vi "GetShiftTime.vi"(8 "error in (no error)":errorcluster, 11 "Time":timestamp) -> (0 "error out":errorcluster, 1 "Shift Elapsed Time [s]":dbl, 2 "Shift Start Time":timestamp, 3 "Shift End Time":timestamp)   [LabVIEW 2016]
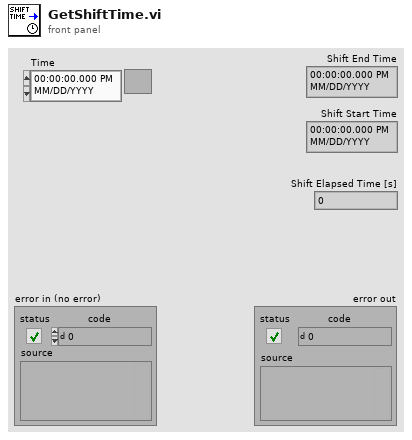
[diagram p1: front panel]
types:
  T1 = typedef "LVDateTimeRec.ctl" = cluster{"fractional second":dbl, "second":i32, "minute":i32, "hour":i32, "day of month":i32, "month":i32, "year":i32, "day of week":i32, "day of year":i32, "DST":i32}
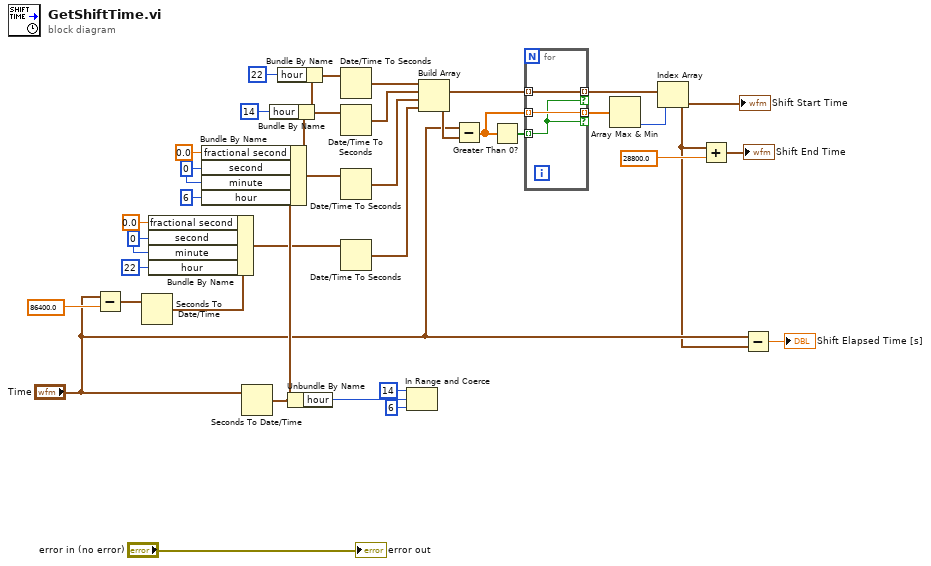
[diagram p0: block diagram]
diagram:
  w12 = 0 ("second")
  w31 = 0 ("second")
  n1 = Subtract(x="Time", y=86400.0 ("fractional second")) -> (x-y=w14:timestamp)
  n2 = Seconds To Date/Time(time stamp (now)=w14) -> (date time rec=w10:T1)  [unwired: 1 in]
  n3 = Bundle By Name(cluster=w10, "fractional second"=0.0, "second"=w12, "minute"=w12, "hour"=22) -> (w9:T1)
  n4 = Seconds To Date/Time(time stamp (now)="Time") -> (date time rec=w30:T1)  [unwired: 1 in]
  n5 = Bundle By Name(cluster=w30, "fractional second"=0.0, "second"=w31, "minute"=w31, "hour"=6) -> (w26:T1)
  n6 = Bundle By Name(cluster=w26, "hour"=14) -> (w25:T1)
  n7 = Bundle By Name(cluster=w25, "hour"=22) -> (w24:T1)
  n8 = Unbundle By Name(w30) -> ("hour"=w34:i32)
  n9 = Date/Time To Seconds(2:w24) -> (0:w23:timestamp)  [unwired: 1 in]
  n10 = Date/Time To Seconds(2:w25) -> (0:w22:timestamp)  [unwired: 1 in]
  n11 = Date/Time To Seconds(2:w26) -> (0:w21:timestamp)  [unwired: 1 in]
  n12 = Date/Time To Seconds(2:w9) -> (0:w8:timestamp)  [unwired: 1 in]
  n13 = In Range and Coerce(upper limit=14, x=w34, lower limit=6) -> ()  [unwired: 2 out]
  n14 = Build Array(w23, w22, w21, w8) -> (w20:timestamp[])
  n15 = Subtract(x="Time", y=w20) -> (x-y=w5:dbl[])
  n16 = Greater Than 0?(x=w5) -> (x > 0?=w19:bool[])
  n17 = for {
    tunnel: w20 -> [w38] mode=indexing
    tunnel: [w38] -> w18 mode=indexing if=w36
    tunnel: w19 -> [w36] mode=indexing
    tunnel: [w37] -> w17 mode=indexing if=w36
    tunnel: w5 -> [w37] mode=indexing
  }
  n18 = Array Max & Min(array=w17) -> (min index (indices)=w16:i32)  [unwired: 3 out]
  n19 = Index Array(array=w18, index=w16) -> (element=w3:timestamp)
  "Shift Start Time" <- w3
  n20 = Add(x=w3, y=28800.0 ("fractional second")) -> (x+y=→"Shift End Time":timestamp)
  n21 = Subtract(x="Time", y=w3) -> (x-y=→"Shift Elapsed Time [s]":dbl)
  "error out" <- "error in (no error)"
